vi "Stepper Configure.vi"(6 "Control Method":u8(ring)=1 items=["2 Wire (Pulse & Direction)"=1, "2 Wire"=2, "4 Wire"=4, "EasyDriver"=6, "AF Motor Shield (Stepper 1 & 2 Only)"=5], 7 "Stepper #":u8, 8 "error in":errorcluster, 10 "Stepper Pins":u8[](array[numeric])=[2, 3], 11 "Arduino Resource":T1={"VISA resource"="", "Board Type"=enum."Arduino Uno", "Connection Type"=enum."USB / Serial", "Bytes Per Packet (15)"=15}) -> (0 "error out":errorcluster, 3 "Arduino Resource Out":T1={"VISA resource"="", "Board Type"=enum."Arduino Uno", "Connection Type"=enum."USB / Serial", "Bytes Per Packet (15)"=15})   [LabVIEW 2011, in "LabVIEW Interface for Arduino.lvlib"]
doc: "Specify a stepper #(0-7) and the digital pins for H-bridge based or step & direction stepper drivers. Specify a stepper #(0-1) without pins for use with the Adafruit Motor Shield."
uses:
  <vilib>/LabVIEW Interface for Arduino/LabVIEW Interface for Arduino.lvlib
  <vilib>/LabVIEW Interface for Arduino/Private/Type Defs/Arduino Resource.ctl
  <vilib>/LabVIEW Interface for Arduino/Private/Type Defs/Board Type.ctl
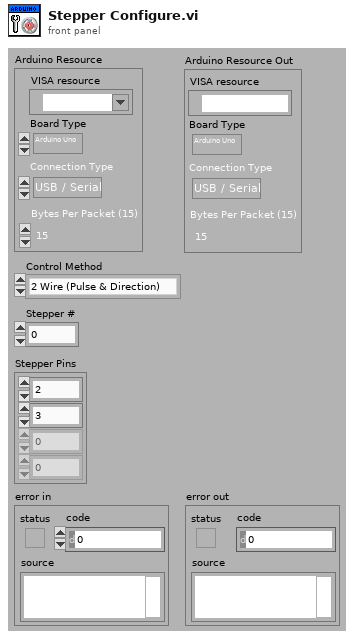
[diagram p1: front panel]
types:
  T1 = typedef "LabVIEW Interface for Arduino.lvlib/Arduino Resource.ctl" = cluster{"VISA resource":refnum<visa-resource-name>, "Board Type":T2, "Connection Type":enum8{"USB / Serial"}, "Bytes Per Packet (15)":u8}
  T2 = typedef "LabVIEW Interface for Arduino.lvlib/Board Type.ctl" = enum16{"Arduino Uno", "Dimuelanove w/Atmega 328", "Mega 2560", "Chipkit Uno32", "Chipkit Max32"}
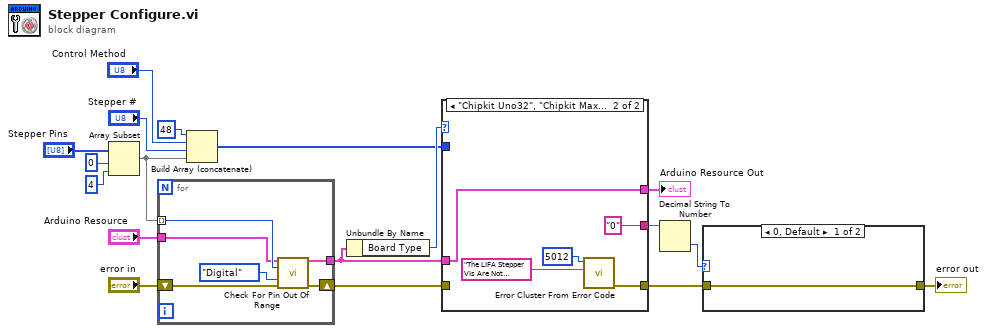
[diagram p0: block diagram]
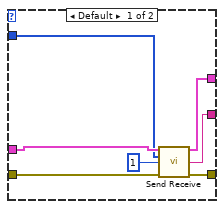
[diagram p2: hidden frame]
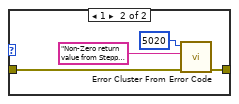
[diagram p3: hidden frame]
diagram:
  n1 = Array Subset(array="Stepper Pins", index=0, length=4) -> (w10:u8[])
  n2 = for {
    tunnel: w10 -> [w24] mode=indexing
    tunnel: "Arduino Resource" -> [w22]
    tunnel: [w21] -> w3
    shift-right: [w19] -> w1
    shift-left: "error in" -> [w20]
    n3 = call <vilib>:"Check For Pin Out Of Range.vi"("Arduino Resource"=w22, "User Pin Number"=w24, "Pin Type"=enum16{"Analog", "Digital"}."Digital", "error in"=w20) -> ("Arduino Resource"=w21:T1, "error out"=w19:errorcluster)  [unwired: 10 in]
  }
  n4 = Build Array (concatenate)(u8 48, "Control Method", "Stepper #", w10) -> (w6:u8[])
  n5 = Unbundle By Name(w3) -> ("Board Type"=w7:T2)
  n6 = case shown="\"Chipkit Uno32\", \"Chipkit Max32\"" w7 {
    tunnel: [w29 w34] -> w4
    tunnel: w3 -> [w30 w33]
    tunnel: w6 -> [w28 _]
    tunnel: [w27 w33] -> w5
    tunnel: [w26 "0" ("Read Buffer")] -> w2
    tunnel: w1 -> [w25 _]
    frame Default {
      n7 = call <vilib>:"Send Receive.vi"("Arduino Resource"=w30, "Data"=w28, "Bytes To Read (0)"=u8 1, "error in"=w25) -> ("Arduino Resource"=w27:T1, "Read Buffer"=w26:string, "error out"=w29:errorcluster)  [unwired: 9 in]
    }
    frame "Chipkit Uno32", "Chipkit Max32" {
      n8 = call <vilib>:"Error Cluster From Error Code.vi"("error message (\"\")"="The LIFA Stepper VIs Are Not Supported On Chipkit Targets." ("source"), "error code (0)"=5012) -> ("error out"=w34:errorcluster)  [unwired: 7 in]
    }
  }
  "Arduino Resource Out" <- w5
  n9 = Decimal String To Number(string=w2) -> (number=w8:i32)  [unwired: 2 in, 1 out]
  n10 = case shown="0, Default" w8 {
    tunnel: w4 -> [w37 w39]
    tunnel: [w37 w38] -> w9
    frame 0, Default {
    }
    frame 1 {
      n11 = call <vilib>:"Error Cluster From Error Code.vi"("error in (no error)"=w39, "error message (\"\")"="Non-Zero return value from Stepper Configure" ("source"), "error code (0)"=5020) -> ("error out"=w38:errorcluster)  [unwired: 6 in]
    }
  }
  "error out" <- w9
